vi "Get Class Paths from Packed Project Library.vi"(8 "error in (no error)":errorcluster, 11 "Packed Library Path":path) -> (0 "error out":errorcluster, 3 "Class List[]":path[](array[path]))   [LabVIEW 2016, in "SLL Class.lvlib"]
doc: "Get list of classes present inside LabVIEW Packed Project Library (PPLs)"
uses:
  SLL Class.lvlib
  <vilib>/Utility/LVLibp/NI_PackedLibraryUtility.lvlib
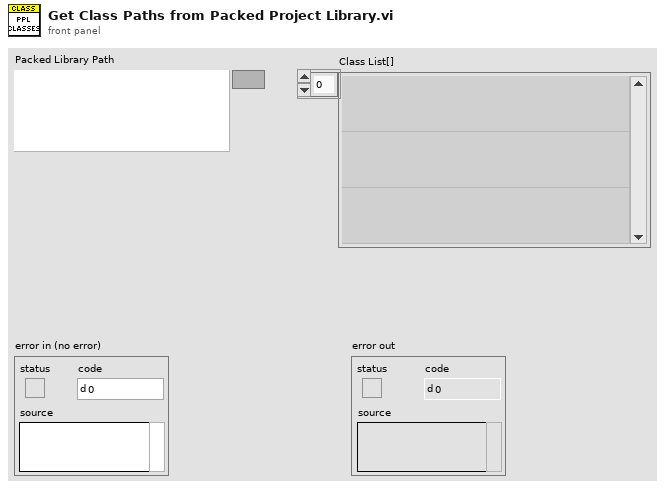
[diagram p1: front panel]
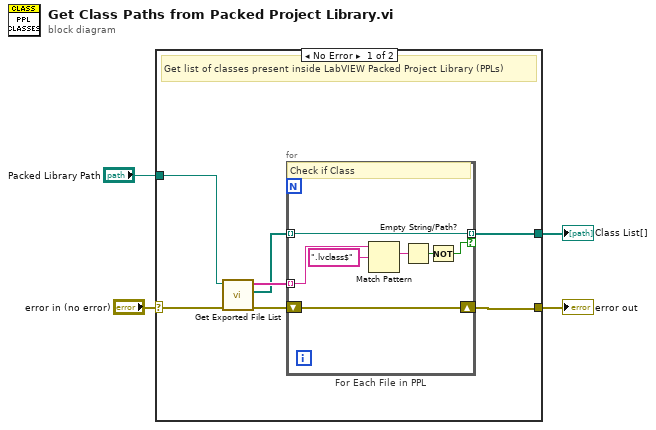
[diagram p0: block diagram]
diagram:
  n1 = case shown="No Error" "error in (no error)" {
    selector: "error in (no error)" -> [w6 w19]
    tunnel: [w11 w19] -> w3
    tunnel: "Packed Library Path" -> [w7 _]
    tunnel: [w5 _] -> w1
    frame No Error {
      # "Get list of classes present inside LabVIEW Packed Project Library (PPLs)"
      n2 = call <vilib>:"Get Exported File List.vi"("error in (no error)"=w6, "packed library path"=w7) -> ("error out"=w10:errorcluster, "paths"=w8:path[], "qualified names"=w9:string[])  [unwired: 7 in]
      n3 = for "For Each File in PPL" {
        tunnel: w9 -> [w18] mode=indexing
        tunnel: w8 -> [w14] mode=indexing
        tunnel: [w14] -> w5 mode=indexing if=w12
        shift-right: [w13] -> w11
        shift-left: w10 -> [w13]
        # "Check if Class"
        n4 = Match Pattern(string=w18, regular expression=".lvclass$") -> (match substring=w16:string)  [unwired: 1 in, 3 out]
        n5 = Empty String/Path?(string/path=w16) -> (empty?=w15:bool)
        n6 = Not(x=w15) -> (.not. x?=w12:bool)
      }
    }
    frame Error {
    }
  }
  "error out" <- w3
  "Class List[]" <- w1
